vi "SMC_GetAI.vi"(8 "error in (no error)":errorcluster) -> (0 "error out":errorcluster, 1 "Average Value":dbl format="%.6f", 2 "Output in Volts":dbl format="%.6f", 3 "Answer":string)   [LabVIEW 2015]
uses:
  SMC_SubVIs.llb/SMC_ManagerMode.ctl
  <vilib>/Analysis/baseanly.llb/Mean (DBL).vi
  <vilib>/Analysis/NI_AALBase.lvlib
panel:
  in  "Scaling factor":dbl=0.000353295 format="%.10f"
  in  "Offset":dbl=140.0 format="%.2f"
  out "Waveform Chart":cluster{"mean":dbl, "mean":dbl}(graph)
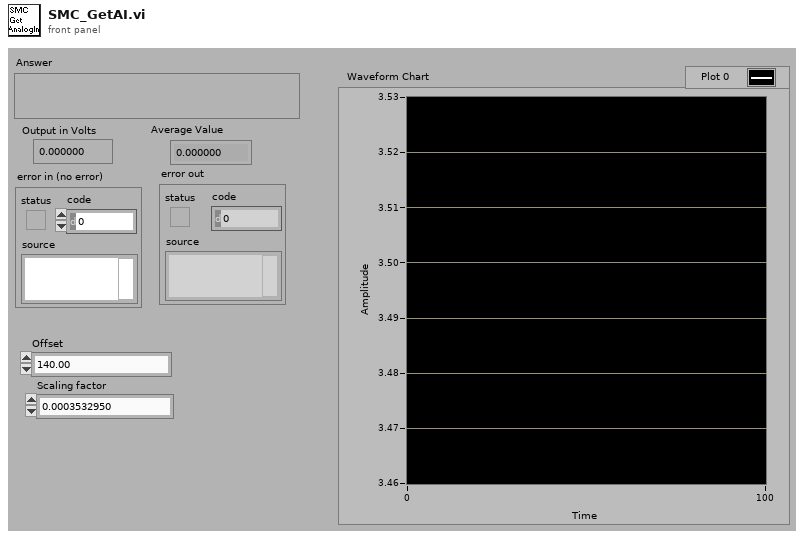
[diagram p1: front panel]
types:
  T1 = typedef "SMC_ManagerMode.ctl" = enum16{"Init", "Get", "SetPosition", "SetStatus", "SetMoving", "SetControllerNr"}
  T2 = typedef "SMC Paras.ctl" = cluster{"VENUS Language":T3, "Number of Axis":u8, "Controller Nr":u8, "Simulation":bool}
  T3 = typedef "VENUSNr.ctl" = enum16{"VENUS 2", "VENUS 1"}
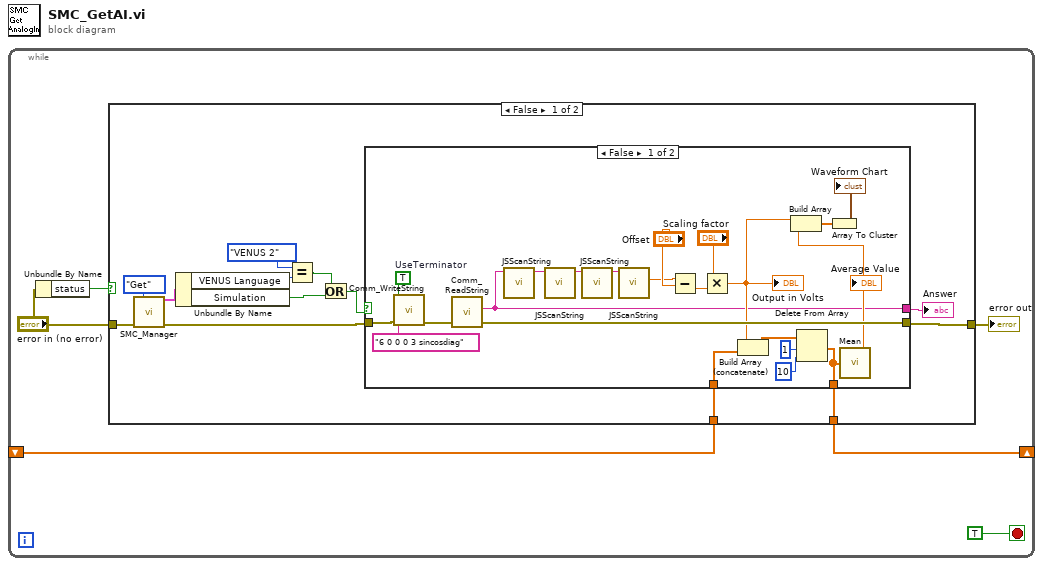
[diagram p0: block diagram]
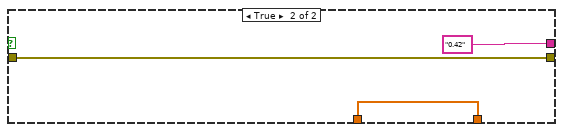
[diagram p2: hidden frame]
diagram:
  n1 = while {
    shift-right: [w1] -> _
    shift-left: _ -> [w2]
    stop <- TRUE stop-if-true
    n2 = Unbundle By Name("error in (no error)") -> ("status"=w6:bool)
    n3 = case shown="False" w6 {
      tunnel: "error in (no error)" -> [w18 w46]
      tunnel: [w15 w46] -> w4
      tunnel: w2 -> [w14 w45]
      tunnel: [w13 w45] -> w1
      frame False {
        n4 = call "SMC_Manager.vi"("Mode"=SMC_ManagerMode."Get", "error in (no error)"=w18) -> ("SMC Parameter Out"=w8:T2, "error out"=w16:errorcluster)  [unwired: 9 in, 3 out]
        n5 = Unbundle By Name(w8) -> ("VENUS Language"=w9:T3, "Simulation"=w7:bool)
        n6 = Equal?(x=enum16{"VENUS 2", "VENUS 1"}."VENUS 2", y=w9) -> (x = y?=w10:bool)
        n7 = Or(x=w10, y=w7) -> (x .or. y?=w11:bool)
        n8 = case shown="False" w11 {
          tunnel: [w23 "0.42" ("Answer")] -> w17
          tunnel: w16 -> [w40 w44]
          tunnel: [w38 w44] -> w15
          tunnel: w14 -> [w26 w42]
          tunnel: [w28 w42] -> w13
          frame False {
            w20 = TRUE  # UseTerminator
            n9 = call "Comm_WriteString.vi"("string to write"="6 0 0 0 3 sincosdiag", "error in (no error)"=w40, "UseTerminator"=w20) -> ("error out"=w39:errorcluster)  [unwired: 8 in]
            n10 = call "Comm_ReadString.vi"("error in (no error)"=w39) -> ("error out"=w38:errorcluster, "Answer"=w23:string)  [unwired: 9 in]
            n11 = call "JSScanString.vi"("String"=w23) -> ("String Out"=w25:string)  [unwired: 9 in, 1 out]
            n12 = call "JSScanString.vi"("String"=w25) -> ("String Out"=w24:string)  [unwired: 9 in, 1 out]
            n13 = call "JSScanString.vi"("String"=w24) -> ("String Out"=w22:string)  [unwired: 9 in, 1 out]
            n14 = call "JSScanString.vi"("String"=w22) -> ("result"=w21:dbl)  [unwired: 9 in, 1 out]
            n15 = Subtract(x=w21, y="Offset") -> (x-y=w37:dbl)
            n16 = Multiply(x="Scaling factor", y=w37) -> (x*y=w27:dbl)
            "Output in Volts" <- w27
            n17 = Build Array (concatenate)(w27, w26) -> (w29:dbl[])
            n18 = Delete From Array(array=w29, length=1 ("Length"), index=10 ("Index")) -> (array with subset deleted=w28:dbl[])  [unwired: 1 out]
            n19 = call-poly <vilib>:"Mean.vi"("X"=w28) -> ("mean"=w31:dbl)  [unwired: 1 out]
            "Average Value" <- w31
            n20 = Build Array(w27, w31) -> (w32:dbl[])
            n21 = Array To Cluster(array=w32) -> (cluster=→"Waveform Chart":cluster{"[0]":dbl, "[1]":dbl})
          }
          frame True {
          }
        }
        "Answer" <- w17
      }
      frame True {
        # "Error, do nothing"
      }
    }
    "error out" <- w4
  }
